vi "Cache_Info Global_Write.vi"(9 "Is Interface?":bool, 10 "Class Info":T1, 11 "Class Name":string) -> ()   [LabVIEW 2019, in "ClassLoader.lvlib"]
uses:
  ClassLoader.lvlib
  Cache_Info Global.vi
  Ctl/Ctl_Class Info.ctl
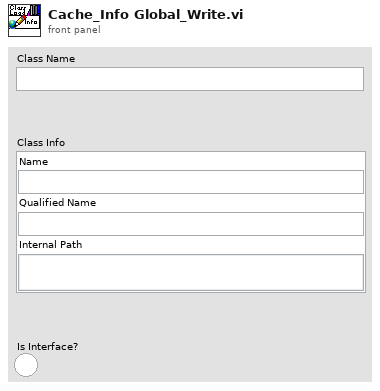
[diagram p1: front panel]
types:
  T1 = typedef "ClassLoader.lvlib/Ctl_Class Info.ctl" = cluster{"Name":string, "Qualified Name":string, "Internal Path":string}
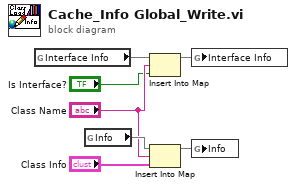
[diagram p0: block diagram]
diagram:
  n1 = global read "Cache_Info Global.vi" "Interface Info"() -> (w4:map{string, bool})
  n2 = global read "Cache_Info Global.vi" "Info"() -> (w7:map{string, T1})
  n3 = Insert Into Map(map in=w4, key="Class Name", value="Is Interface?") -> (map out=w5:map{string, bool})  [unwired: 2 out]
  n4 = Insert Into Map(map in=w7, key="Class Name", value="Class Info") -> (map out=w6:map{string, T1})  [unwired: 2 out]
  n5 = global write "Cache_Info Global.vi" "Interface Info"(w5) -> ()
  n6 = global write "Cache_Info Global.vi" "Info"(w6) -> ()
